vi "Apply Schedule Core.vi"(8 "error in (no error)":errorcluster, 9 "Settings":string, 10 "Schedule":u16(ring) items=["Constant", "Ramp", "Function", "Formula"], 11 "Tool Path in":refnum<class "Tool Path.lvclass">) -> (0 "error out":errorcluster, 2 "Schedule Array":dbl[](array[numeric]), 3 "Tool Path out":refnum<class "Tool Path.lvclass">)   [LabVIEW 2019, in "Tool Path.lvclass"]
uses:
  Tool Path.lvclass
  subVIs/typedefs/Schedule Types/Schedule--Constant.ctl
  Settings/ObjectSettings/ObjectSettings.lvclass
  subVIs/typedefs/Schedule Types/Schedule--Ramp.ctl
  <vilib>/Analysis/NI_AALBase.lvlib
  subVIs/typedefs/Schedule Types/Schedule--Function Generator.ctl
  <vilib>/measure/NI_MABase.lvlib
  subVIs/typedefs/Schedule Types/Schedule--Formula.ctl
  <vilib>/gmath/NI_Gmath.lvlib
  subVIs/typedefs/Schedule - enum.ctl
  <vilib>/Analysis/1siggen.llb/Ramp Pattern by Samples.vi
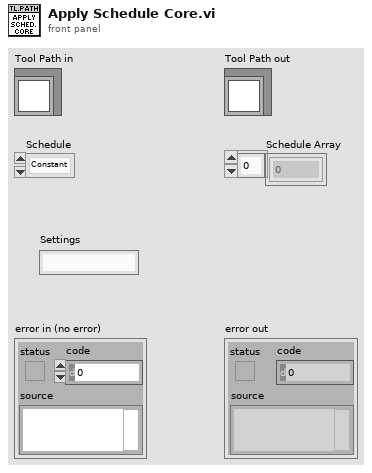
[diagram p1: front panel]
types:
  T1 = typedef "Schedule - enum.ctl" = enum16{"Constant", "Ramp", "Fn. Generator", "Formula"}
  T2 = enum16{"Sine Wave", "Triangle Wave", "Square Wave", "Sawtooth Wave"}
  T3 = typedef "Schedule--Constant.ctl" = cluster{"Value":dbl}
  T4 = typedef "Schedule--Ramp.ctl" = cluster{"Start":dbl, "End":dbl}
  T5 = typedef "Schedule--Function Generator.ctl" = cluster{"Min Value":dbl, "Max Value":dbl, "Duty Cycle (%)":dbl, "Signal Type":u16, "Cycle Number":dbl, "Phase (degrees)":dbl}
  T6 = typedef "Schedule--Formula.ctl" = cluster{"formula":string, "formula length (nm)":dbl, "formula resolution (nm)":dbl}
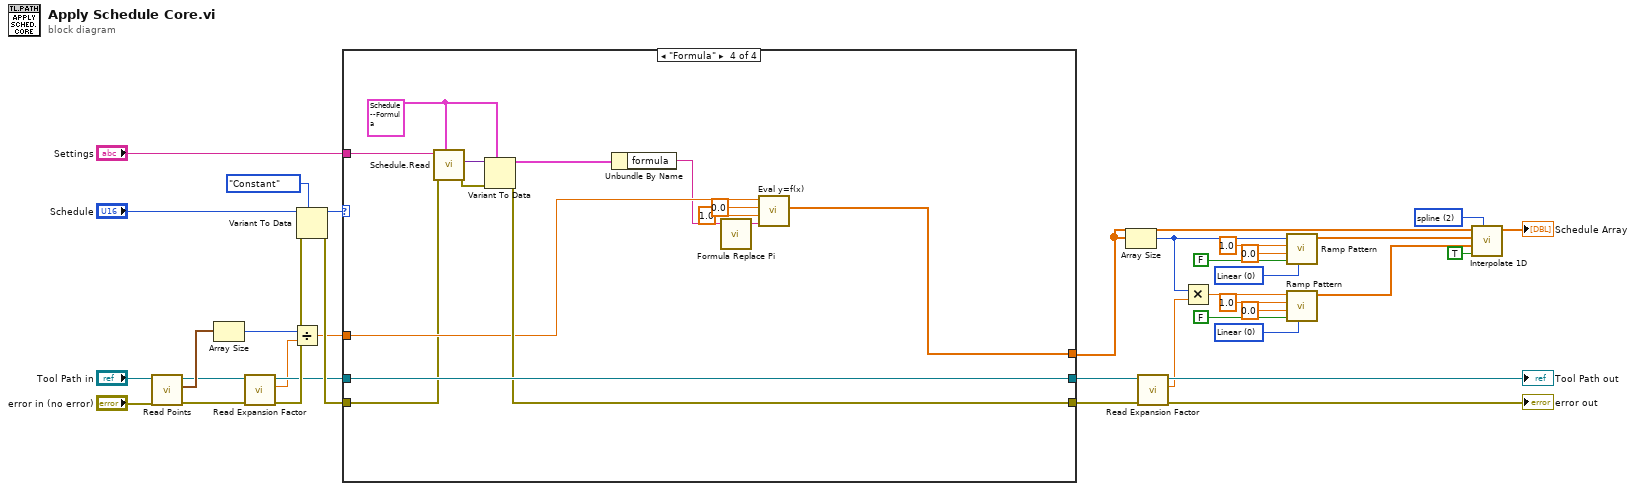
[diagram p0: block diagram]
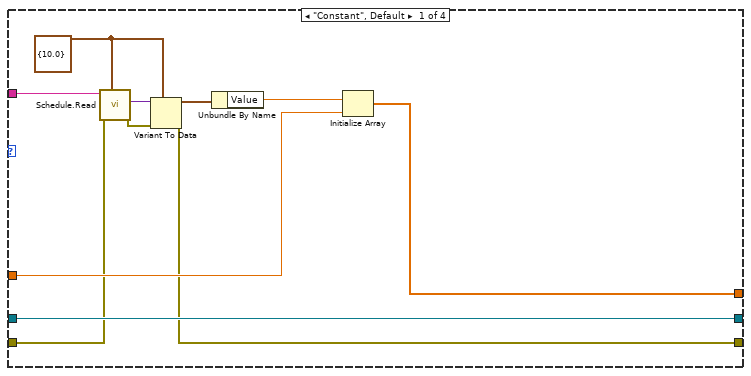
[diagram p2: hidden frame]
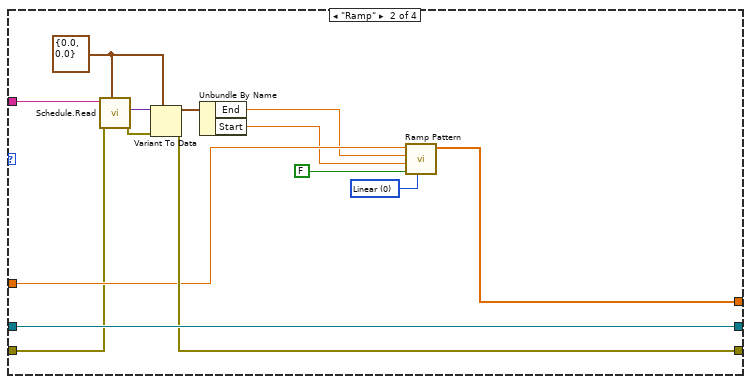
[diagram p3: hidden frame]
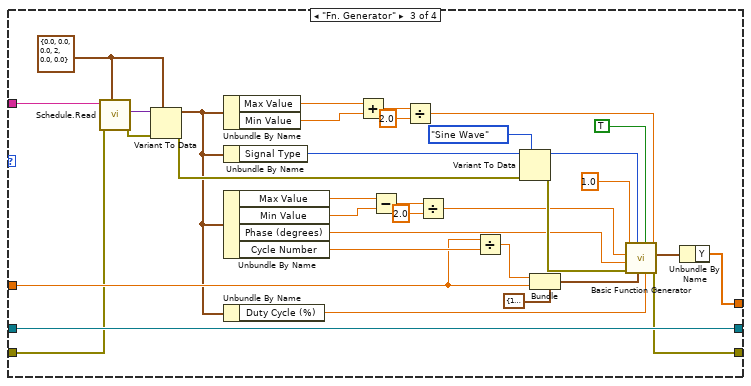
[diagram p4: hidden frame]
diagram:
  w9 = u16 0 items=["Linear", "Logarithmic"] ("type")
  w19 = u16 0 items=["Linear", "Logarithmic"] ("type")
  w20 = 2 items=["nearest", "linear", "spline", "cubic Hermite", "Lagrange"] ("method")
  n1 = call-dynamic "Read Points.vi"("error in (no error)"="error in (no error)", "Tool Object in"="Tool Path in") -> ("error out"=w27:errorcluster, "Points"=w33:cluster{"X":dbl, "Y":dbl}[], "Tool Object out"=w28:refnum<class "Tool Path.lvclass">)  [unwired: 7 in]
  n2 = Array Size(array=w33) -> (size(s)=w23:i32)
  n3 = call-dynamic "Read Expansion Factor.vi"("error in (no error)"=w27, "Tool Path in"=w28) -> ("error out"=w26:errorcluster, "Expansion Factor"=w22:dbl, "Tool Path out"=w25:refnum<class "Tool Path.lvclass">)  [unwired: 7 in]
  n4 = Divide(x=w23, y=w22) -> (x/y=w24:dbl)
  n5 = Variant To Data(error in=w26, type=Schedule_-_enum."Constant" ("Schedule"), Variant="Schedule") -> (data=w35:T1, error out=w34:errorcluster)
  n6 = case shown="\"Formula\"" w35 {
    tunnel: w25 -> [w47 w61 w95 w109]
    tunnel: [w47 w61 w95 w109] -> w15
    tunnel: w34 -> [w37 w48 w62 w98]
    tunnel: [w39 w59 w71 w104] -> w13
    tunnel: w24 -> [w41 w57 w72 w101]
    tunnel: [w40 w52 w65 w100] -> w2
    tunnel: "Settings" -> [w38 w49 w63 w99]
    frame "Constant", Default {
      w44 = T3 {"Value"=10.0} ("Constant")
      n7 = call "Schedule.Read.vi"("Data to Read"=w44, "error in (no error)"=w37, "Schedule <JSON> In"=w38) -> ("error out"=w45:errorcluster, "Data Out"=w46:variant)  [unwired: 6 in, 1 out]
      n8 = Variant To Data(error in=w45, type=w44, Variant=w46) -> (data=w43:T3, error out=w39:errorcluster)
      n9 = Unbundle By Name(w43) -> ("Value"=w42:dbl)
      n10 = Initialize Array(w42, w41) -> (w40:dbl[])
    }
    frame "Ramp" {
      w56 = u16 0 items=["Linear", "Logarithmic"] ("type")
      w58 = T4 {"Start"=0.0, "End"=0.0} ("Ramp")
      n11 = call "Schedule.Read.vi"("Data to Read"=w58, "error in (no error)"=w48, "Schedule <JSON> In"=w49) -> ("error out"=w50:errorcluster, "Data Out"=w60:variant)  [unwired: 6 in, 1 out]
      n12 = Variant To Data(error in=w50, type=w58, Variant=w60) -> (data=w55:T4, error out=w59:errorcluster)
      n13 = Unbundle By Name(w55) -> ("End"=w51:dbl, "Start"=w54:dbl)
      n14 = call-poly <vilib>:"Ramp Pattern.vi"("type"=w56, "exclude end?"=FALSE, "start"=w54, "end"=w51, "samples"=w57) -> ("Ramp Pattern"=w52:dbl[])  [unwired: 5 in, 1 out]
    }
    frame "Fn. Generator" {
      w92 = T5 {"Min Value"=0.0, "Max Value"=0.0, "Duty Cycle (%)"=0.0, "Signal Type"=2, "Cycle Number"=0.0, "Phase (degrees)"=0.0} ("Fn. Gen")
      n15 = call "Schedule.Read.vi"("Data to Read"=w92, "error in (no error)"=w62, "Schedule <JSON> In"=w63) -> ("error out"=w94:errorcluster, "Data Out"=w93:variant)  [unwired: 6 in, 1 out]
      n16 = Variant To Data(error in=w94, type=w92, Variant=w93) -> (data=w66:T5, error out=w69:errorcluster)
      n17 = Unbundle By Name(w66) -> ("Max Value"=w73:dbl, "Min Value"=w74:dbl)
      n18 = Unbundle By Name(w66) -> ("Signal Type"=w83:u16)
      n19 = Unbundle By Name(w66) -> ("Max Value"=w79:dbl, "Min Value"=w80:dbl, "Phase (degrees)"=w68:dbl, "Cycle Number"=w87:dbl)
      n20 = Unbundle By Name(w66) -> ("Duty Cycle (%)"=w91:dbl)
      n21 = Add(x=w73, y=w74) -> (x+y=w75:dbl)
      n22 = Subtract(x=w79, y=w80) -> (x-y=w78:dbl)
      n23 = Divide(x=w75, y=2.0) -> (x/y=w81:dbl)
      n24 = Divide(x=w78, y=2.0) -> (x/y=w67:dbl)
      n25 = Divide(x=w72, y=w87) -> (x/y=w89:dbl)
      n26 = Variant To Data(error in=w69, type=T2."Sine Wave" ("signal type"), Variant=w83) -> (data=w85:T2, error out=w70:errorcluster)
      n27 = Bundle(cluster=cluster{"Fs":dbl, "#s":dbl} {"Fs"=1000.0, "#s"=1000.0} ("sampling info"), "Fs"=w89, "#s"=w72) -> (w90:cluster{"Fs":dbl, "#s":dbl})
      n28 = call <vilib>:"Basic Function Generator.vi"("offset"=w81, "square wave duty cycle (%)"=w91, "reset signal"=TRUE, "sampling info"=w90, "signal type"=w85, "error in (no error)"=w70, "phase"=w68, "amplitude"=w67, "frequency"=1.0) -> ("error out"=w71:errorcluster, "signal out"=w64:waveform(dbl))  [unwired: 1 out]
      n29 = Unbundle By Name(w64) -> ("Y"=w65:dbl[])
    }
    frame "Formula" {
      w107 = T6 {"formula"="1*(step(170-t)*cos(0.62831853071*t)+step(t-170)*cos(0.62831853071*(t-170))*(-1))", "formula length (nm)"=340.0, "formula resolution (nm)"=0.001} ("Formula")
      n30 = call "Schedule.Read.vi"("Data to Read"=w107, "error in (no error)"=w98, "Schedule <JSON> In"=w99) -> ("error out"=w108:errorcluster, "Data Out"=w106:variant)  [unwired: 6 in, 1 out]
      n31 = Variant To Data(error in=w108, type=w107, Variant=w106) -> (data=w105:T6, error out=w104:errorcluster)
      n32 = Unbundle By Name(w105) -> ("formula"=w97:string)
      n33 = call "Formula Replace Pi.vi"("Formula In"=w97) -> ("Formula Out"=w96:string)  [unwired: 4 in]
      n34 = call <vilib>:"Eval y=f(x).vi"("formula"=w96, "end"=1.0, "start"=0.0, "number of points"=w101) -> ("Y Values"=w100:dbl[])  [unwired: 3 out]
    }
  }
  n35 = Array Size(array=w2) -> (size(s)=w11:i32)
  n36 = call-dynamic "Read Expansion Factor.vi"("error in (no error)"=w13, "Tool Path in"=w15) -> ("error out"=→"error out":errorcluster, "Expansion Factor"=w10:dbl, "Tool Path out"=→"Tool Path out":refnum<class "Tool Path.lvclass">)  [unwired: 7 in]
  n37 = Multiply(x=w11, y=w10) -> (x*y=w6:dbl)
  n38 = call-poly <vilib>:"Ramp Pattern.vi"("type"=w19, "exclude end?"=FALSE, "start"=0.0, "end"=1.0, "samples"=w11) -> ("Ramp Pattern"=w16:dbl[])  [unwired: 5 in, 1 out]
  n39 = call-poly <vilib>:"Ramp Pattern.vi"("type"=w9, "exclude end?"=FALSE, "start"=0.0, "end"=1.0, "samples"=w6) -> ("Ramp Pattern"=w5:dbl[])  [unwired: 5 in, 1 out]
  n40 = call <vilib>:"Interpolate 1D.vi"("method"=w20, "X is monotonic"=TRUE, "xi"=w5, "X"=w16, "Y"=w2) -> ("yi"=→"Schedule Array":dbl[])  [unwired: 4 in, 2 out]
